vi "parse_image_roslv.vi"(4 "error in":errorcluster, 7 "msg in":string) -> (0 "error out":errorcluster, 1 "image data":T1, 2 "ROS Image":T2, 3 "msg out":string)   [LabVIEW 2014]
doc: "Parses a message into an image"
uses:
  <vilib>/picture/picture.llb/imagedata.ctl
  std_msgs/subs/parse_u32_scalar_roslv.vi
  std_msgs/subs/parse_string_scalar_roslv.vi
  std_msgs/subs/parse_u8_scalar_roslv.vi
  std_msgs/subs/parse_u8_array_roslv.vi
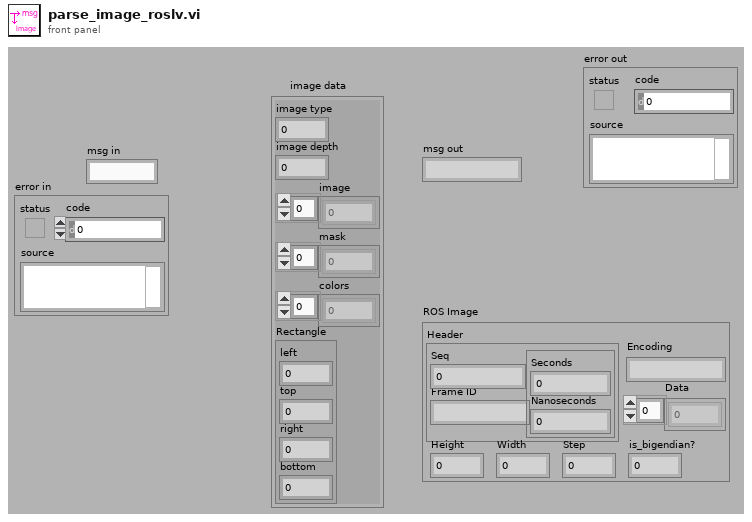
[diagram p1: front panel]
types:
  T1 = typedef "imagedata.ctl" = cluster{"image type":i32, "image depth":i32, "image":u8[], "mask":u8[], "colors":u32[], "Rectangle":cluster{"left":i16, "top":i16, "right":i16, "bottom":i16}}
  T2 = cluster{"Header":cluster{"Seq":u32, "Frame ID":string, cluster{"Seconds":i32, "Nanoseconds":i32}}, "Height":u32, "Width":u32, "is_bigendian?":u8, "Step":u32, "Data":u8[], "Encoding":string}
  T3 = cluster{"Seq":u32, "Frame ID":string, "Timestamp":cluster{"Seconds":i32, "Nanoseconds":i32}}
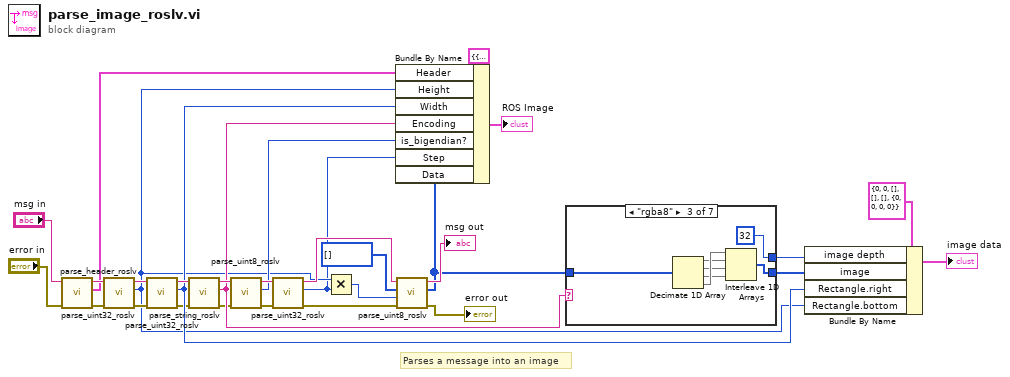
[diagram p0: block diagram]
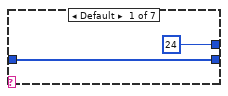
[diagram p2: hidden frame]
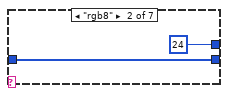
[diagram p3: hidden frame]
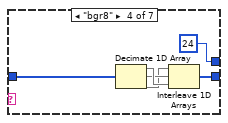
[diagram p4: hidden frame]
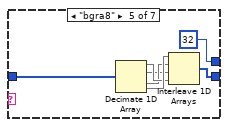
[diagram p5: hidden frame]
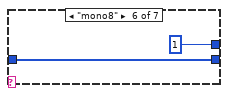
[diagram p6: hidden frame]
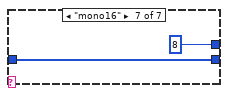
[diagram p7: hidden frame]
diagram:
  # "Parses a message into an image"
  n1 = call "parse_header_roslv.vi"("error in"="error in", "msg in"="msg in") -> ("error out"=w10:errorcluster, "Header"=w23:T3, "msg out"=w31:string)  [unwired: 3 in]
  n2 = call-poly "parse_uint32_roslv.vi"("error in"=w10, "msg in"=w31) -> ("error out"=w11:errorcluster, "number"=w4:u32, "msg out"=w30:string)  [unwired: 3 in]
  n3 = call-poly "parse_uint32_roslv.vi"("error in"=w11, "msg in"=w30) -> ("error out"=w12:errorcluster, "number"=w16:u32, "msg out"=w29:string)  [unwired: 3 in]
  n4 = call-poly "parse_string_roslv.vi"("error in"=w12, "msg in"=w29) -> ("error out"=w13:errorcluster, "string"=w19:string, "msg out"=w28:string)  [unwired: 3 in]
  n5 = call-poly "parse_uint8_roslv.vi"("error in"=w13, "msg in"=w28) -> ("error out"=w14:errorcluster, "number"=w22:u8, "msg out"=w27:string)  [unwired: 3 in]
  n6 = call-poly "parse_uint32_roslv.vi"("error in"=w14, "msg in"=w27) -> ("error out"=w15:errorcluster, "number"=w3:u32, "msg out"=w26:string)  [unwired: 3 in]
  n7 = Multiply(x=w4, y=w3) -> (x*y=w1:u32)
  n8 = call-poly "parse_uint8_roslv.vi"("error in"=w15, "Array Size"=w1, "type"=u8[] [], "msg in"=w26) -> ("error out"=→"error out":errorcluster, "number"=w20:u8[], "msg out"=→"msg out":string)  [unwired: 1 in]
  n9 = Bundle By Name(cluster=T2 {"Header"={"Seq"=0, "Frame ID"="", {"Seconds"=0, "Nanoseconds"=0}}, "Height"=0, "Width"=0, "is_bigendian?"=0, "Step"=0, "Data"=[], "Encoding"=""} ("ROS Image"), "Header"=w23, "Height"=w4, "Width"=w16, "Encoding"=w19, "is_bigendian?"=w22, "Step"=w3, "Data"=w20) -> (→"ROS Image":T2)
  n10 = case shown="\"rgba8\"" w19 {
    tunnel: w20 -> [w33 w35 w41 w48 w55 w57 w59]
    tunnel: [w33 w35 w40 w47 w54 w57 w59] -> w17
    tunnel: [24 ("Depth") 24 ("Depth") 32 ("Depth") 24 ("Depth") 32 ("Depth") 1 ("Depth") 8 ("Depth")] -> w18
    frame Default {
    }
    frame "rgb8" {
    }
    frame "rgba8" {
      n11 = Decimate 1D Array(w41) -> (w38:u8[], w37:u8[], w36:u8[], w39:u8[])
      n12 = Interleave 1D Arrays(w39, w38, w37, w36) -> (w40:u8[])
    }
    frame "bgr8" {
      n13 = Decimate 1D Array(w48) -> (w46:u8[], w45:u8[], w44:u8[])
      n14 = Interleave 1D Arrays(w44, w45, w46) -> (w47:u8[])
    }
    frame "bgra8" {
      n15 = Decimate 1D Array(w55) -> (w51:u8[], w49:u8[], w50:u8[], w52:u8[])
      n16 = Interleave 1D Arrays(w52, w50, w49, w51) -> (w54:u8[])
    }
    frame "mono8" {
    }
    frame "mono16" {
    }
  }
  n17 = Bundle By Name(cluster=T1 {"image type"=0, "image depth"=0, "image"=[], "mask"=[], "colors"=[], "Rectangle"={"left"=0, "top"=0, "right"=0, "bottom"=0}} ("image data"), "image depth"=w18, "image"=w17, "Rectangle.right"=w16, "Rectangle.bottom"=w4) -> (→"image data":T1)
